vi "Fix Folder of Corrupt TDMS files.vi"() -> ()   [LabVIEW 2016]
panel:
  in  "stop":bool
  out "Currently Processing":path
  out "Progress (%)":u8(slide) scale=0.0..100.0
  in  "folder to fix":path
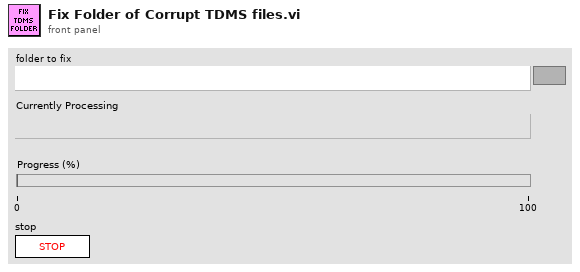
[diagram p1: front panel]
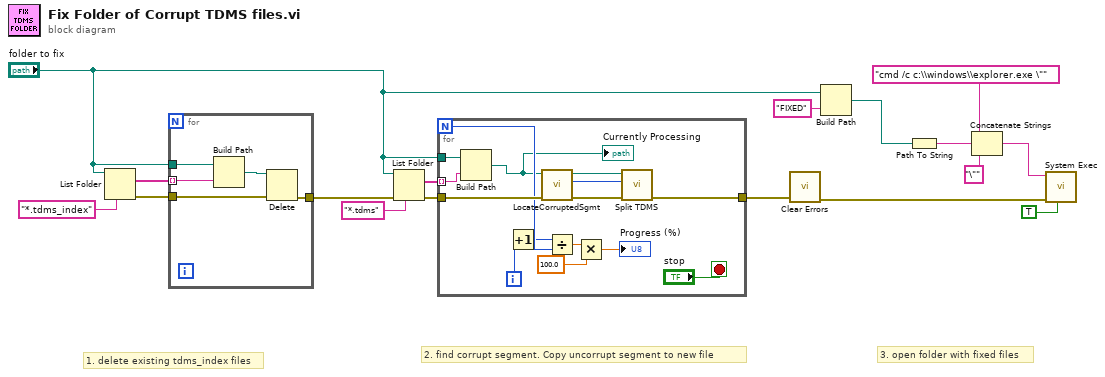
[diagram p0: block diagram]
diagram:
  # "3. open folder with fixed files"
  # "2. find corrupt segment. Copy uncorrupt segment to new file"
  # "1. delete existing tdms_index files"
  n1 = List Folder(path="folder to fix", pattern="*.tdms_index") -> (filenames=w2:string[], error out=w4:errorcluster)  [unwired: 2 in, 2 out]
  n2 = for {
    tunnel: w4 -> [w21]
    tunnel: [w22] -> w3
    tunnel: w2 -> [w19] mode=indexing
    tunnel: "folder to fix" -> [w18]
    n3 = Build Path(base path=w18, name or relative path=w19) -> (appended path=w20:path)
    n4 = Delete(path (use dialog)=w20, error in=w21) -> (error out=w22:errorcluster)  [unwired: 3 in, 2 out]
  }
  n5 = List Folder(path="folder to fix", pattern="*.tdms", error in=w3) -> (filenames=w13:string[], error out=w17:errorcluster)  [unwired: 1 in, 2 out]
  n6 = for {
    N -> [w33]
    tunnel: w17 -> [w37]
    tunnel: [w26] -> w15
    tunnel: w13 -> [w24] mode=indexing
    tunnel: "folder to fix" -> [w25]
    i -> [w32]
    stop <- "stop" stop-if-true
    n7 = Build Path(base path=w25, name or relative path=w24) -> (appended path=w23:path)
    "Currently Processing" <- w23
    n8 = Increment(x=w32) -> (x+1=w27:i32)
    n9 = call "LocateCorruptedSgmt.vi"("error in"=w37, "file path (use dialog)"=w23) -> ("error out"=w36:errorcluster, "corrupted sgmt"=w34:i32, "path"=w35:path)  [unwired: 7 in]
    n10 = Divide(x=w27, y=w33) -> (x/y=w31:dbl)
    n11 = Multiply(x=w31, y=100.0) -> (x*y=→"Progress (%)":dbl)
    n12 = call "Split TDMS.vi"("error in"=w36, "Segments per file"=w34, "file path (use dialog)"=w35) -> ("error out"=w26:errorcluster)  [unwired: 8 in]
  }
  n13 = call <vilib>:"Clear Errors.vi"("error in (no error)"=w15) -> ("error out"=w12:errorcluster)  [unwired: 5 in, 1 out]
  n14 = Build Path(base path="folder to fix", name or relative path="FIXED") -> (appended path=w9:path)
  n15 = Path To String(path=w9) -> (string=w8:string)
  n16 = Concatenate Strings("cmd /c c:\\windows\\explorer.exe \"", w8, "\"") -> (w6:string)
  n17 = call <vilib>:"System Exec.vi"("run minimized? (F)"=TRUE, "error in (no error)"=w12, "command line"=w6) -> ()  [unwired: 5 in, 4 out]
